vi "DAQ Assistant Express.vi"() -> ()   [LabVIEW 2020]
panel:
  out "error out":errorcluster
  out "data":dynamicdata(graph)
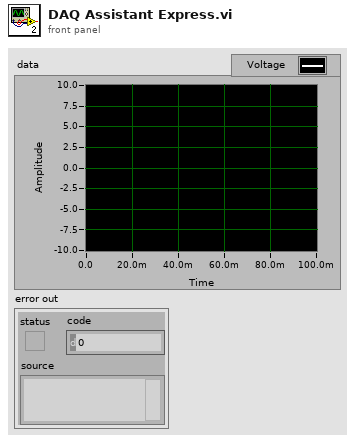
[diagram p1: front panel]
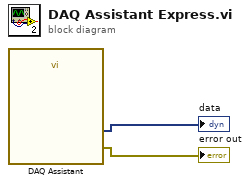
[diagram p0: block diagram]
diagram:
  n1 = call "DAQ Assistant"() -> ("data"=→"data":dynamicdata, "error out"=→"error out":errorcluster)  [unwired: 17 in, 1 out]
